vi "_STL_to_Mesh.vi"() -> ()   [LabVIEW 2026]
uses:
  <vilib>/picture/3D Picture Control/Old 3D Toolkit.llb/model.ctl
  <vilib>/picture/3D Picture Control/Old 3D Toolkit.llb/point3f.ctl
  <vilib>/picture/3D Picture Control/Old 3D Toolkit.llb/VertexMode.ctl
  <vilib>/picture/3D Picture Control/NI_3D Picture Control.lvlib
  <vilib>/picture/3D Picture Control/NI_Old 3D Toolkit.lvlib
panel:
  out "Model Out":T1={"VertexList"=[], "FaceList"=[], "NormalList"=[], "Mode"=enum."GL_TRIANGLES"} {"NormalList"."z" format="%.2f"; "NormalList"."y" format="%.2f"; "NormalList"."x" format="%.2f"; "VertexList"."z" format="%.2f"; "VertexList"."y" format="%.2f"; "VertexList"."x" format="%.2f"}
  in  "Model File":path
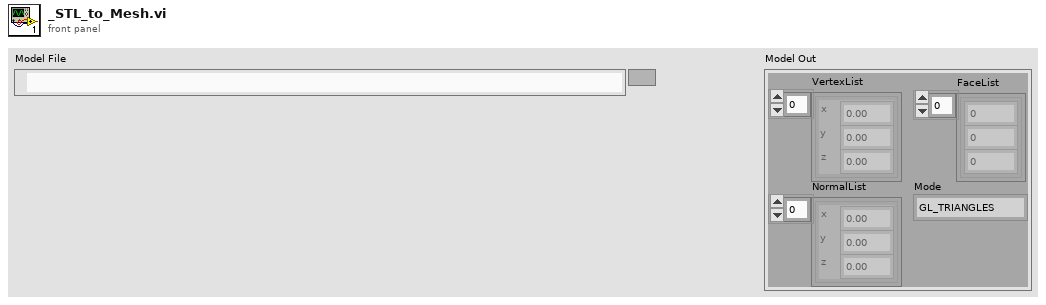
[diagram p1: front panel]
types:
  T1 = typedef "NI_3D Picture Control.lvlib/NI_Old 3D Toolkit.lvlib/model.ctl" = cluster{"VertexList":T2[], "FaceList":cluster{"v1":i32, "v2":i32, "v3":i32}[], "NormalList":T2[], "Mode":T3}
  T2 = typedef "NI_3D Picture Control.lvlib/NI_Old 3D Toolkit.lvlib/point3f.ctl" = cluster{"x":sgl, "y":sgl, "z":sgl}
  T3 = typedef "NI_3D Picture Control.lvlib/NI_Old 3D Toolkit.lvlib/VertexMode.ctl" = enum16{"GL_POINTS", "GL_LINES", "GL_LINE_LOOP", "GL_LINE_STRIP", "GL_TRIANGLES", "GL_TRIANGLE_STRIP", "GL_TRIANGLE_FAN", "GL_QUADS", "GL_QUAD_STRIP", "GL_POLYGON"}
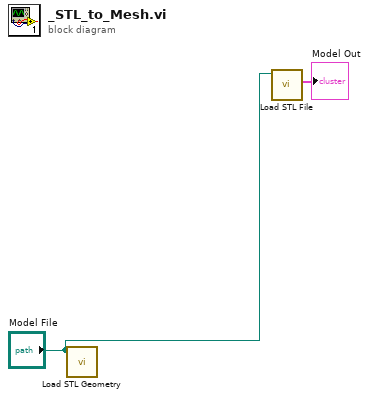
[diagram p0: block diagram]
diagram:
  n1 = call <vilib>:"Load STL Geometry.vi"("Model File"="Model File") -> ()  [unwired: 9 in, 2 out]
  n2 = call <vilib>:"Load STL File.vi"("path to STL file"="Model File") -> ("Model Out"=→"Model Out":T1)  [unwired: 1 in, 9 out]
